vi "stabilizePress_08.vi"() -> ()   [LabVIEW 2011]
uses:
  <vilib>/Analysis/NI_AALPro.lvlib
panel:
  out "Pset array":dbl[](array[numeric])
  out "Pset array":dbl[](array[numeric])
  in  "max plot points":i32=60
  in  "max poly order":u16=2
  out "tune setpoint":dbl=9.864666666660924
  in  "points to fit":i32=4
  out "dt_array":dbl[](array[numeric])
  out "P_i+1 (torr)":dbl caption="predicted next P (torr)" format="%.2f"
  out "Polynomial Coefficients":dbl[](array[numeric])
  in  "polynomial order":dbl=2.0
  out "P array":dbl[](array[numeric])
  out "t array":dbl[](array[numeric])
  in  "i":u16=11
  out "tElaps":dbl=14.796999999991385
  in  "dT_fit(s)":dbl=0.5
  in  "tTotal(s)":dbl=30.0
  out "XY Graph":cluster{"Value":dbl[], "Value":dbl[]}[](graph)
  out "stabilize done":bool
  in  "tExp(s)":dbl=15.0
  out "Set Point (torr)":dbl=20.0 format="%.2f"
  out "Setpoint Index":string="C"
  out "Setpoint Index control":u16(ring)=2 caption="Setpoint" items=["A", "B", "C", "D"]
  out "t_0":dbl=69652.793
  in  "time done (s)":dbl
  out "Wait to set":bool
  out "IO error":errorcluster={"status"=FALSE, "code"=1073676418, "source"="VISA Close in WriteAdaptorr04.vi->writeSetPoint_01.vi->stabilizePress_05.vi"}
  in  "stop":bool=TRUE
  out "Pi (torr)":dbl=6.790000000000001 caption="P(torr)" format="%.2f"
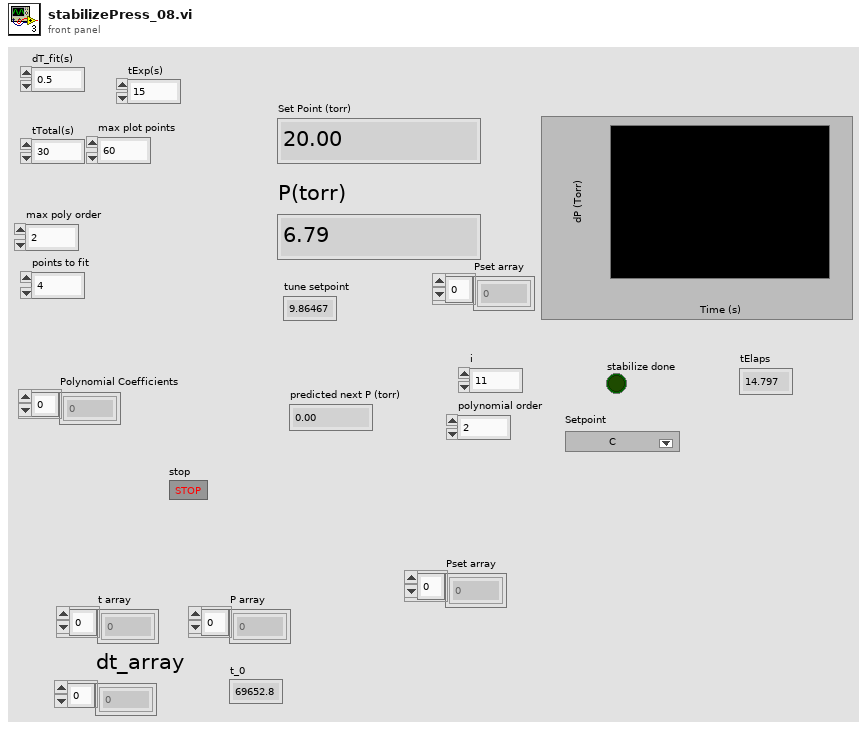
[diagram p1: front panel]
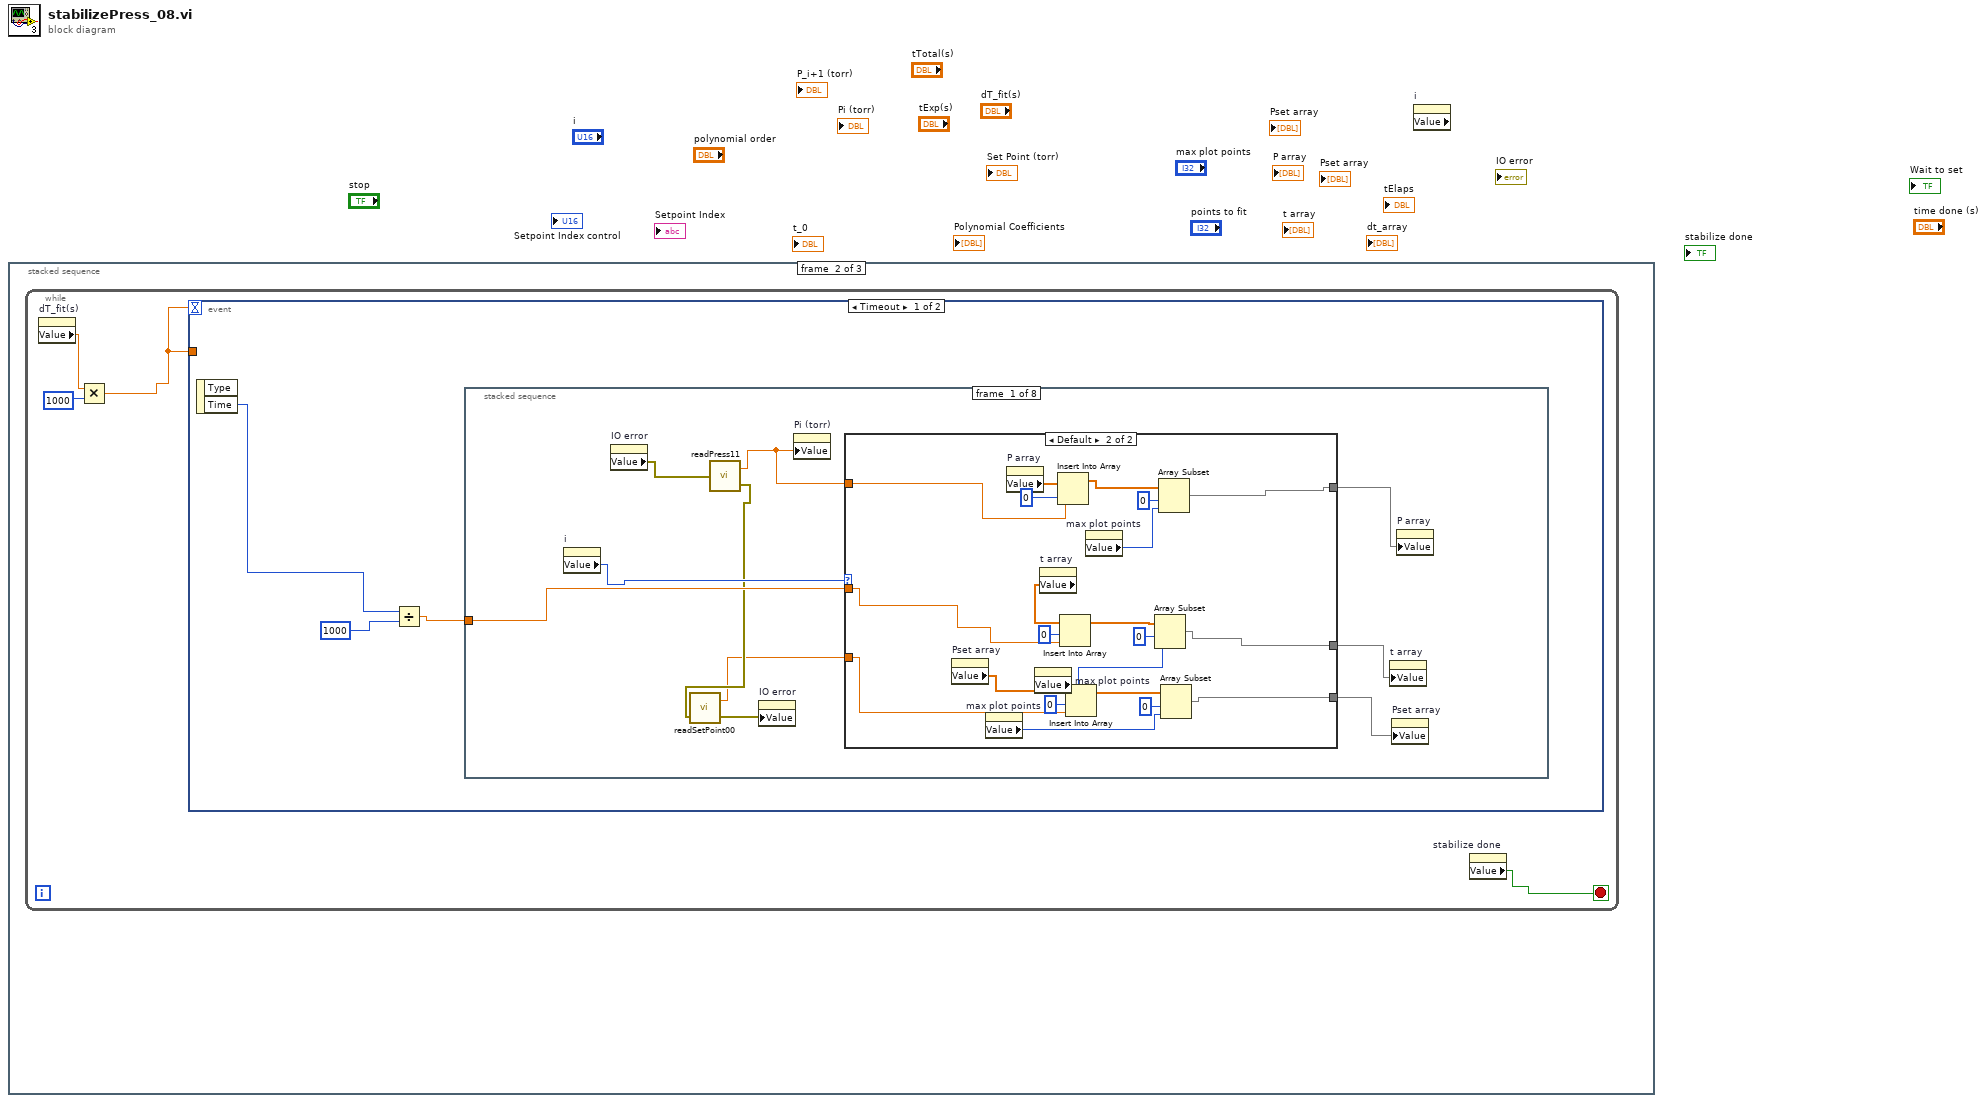
[diagram p0: block diagram]
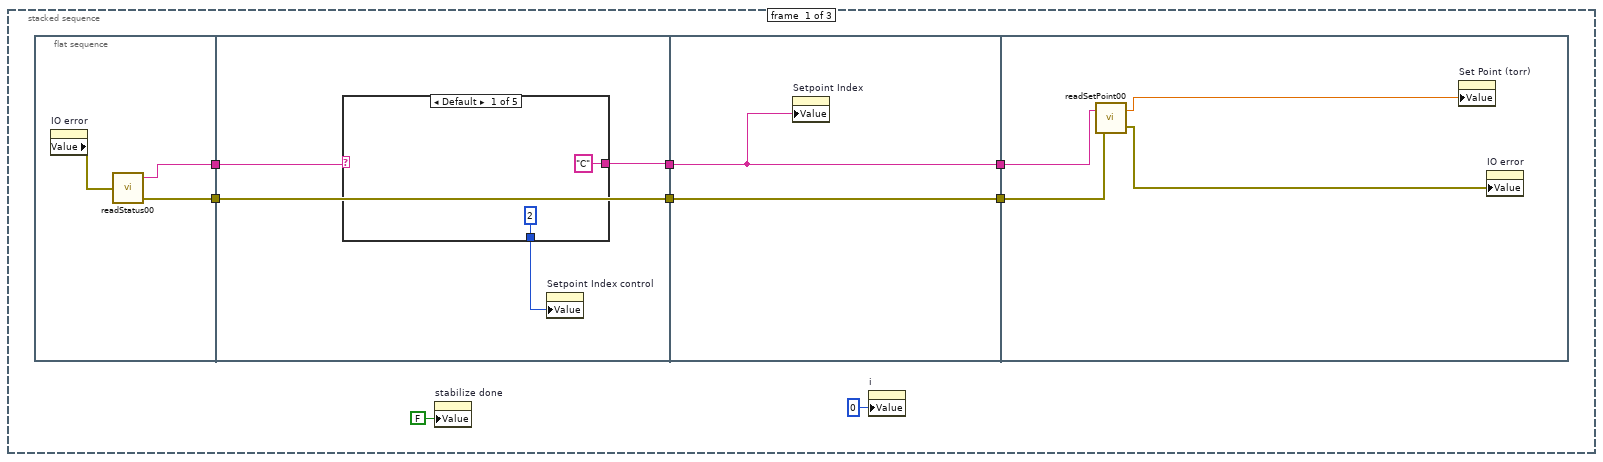
[diagram p2: hidden frame]
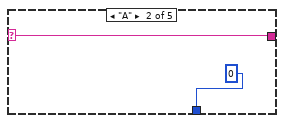
[diagram p3: hidden frame]
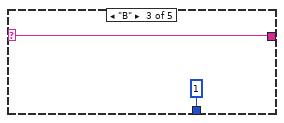
[diagram p4: hidden frame]
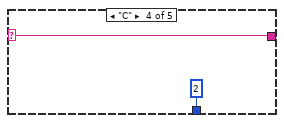
[diagram p5: hidden frame]
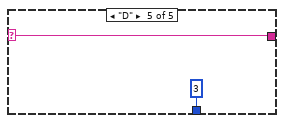
[diagram p6: hidden frame]
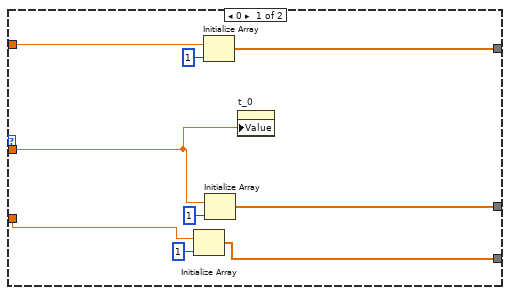
[diagram p7: hidden frame]
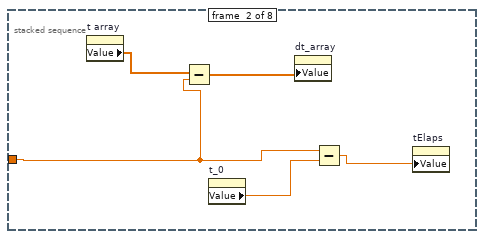
[diagram p8: hidden frame]
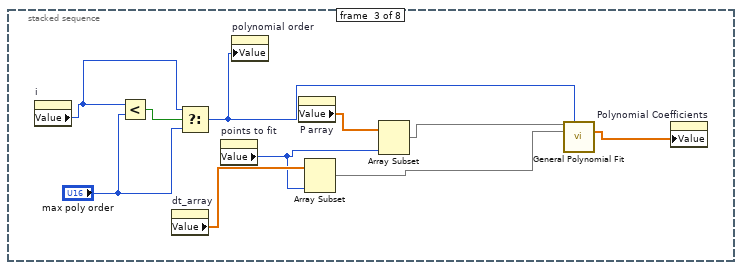
[diagram p9: hidden frame]
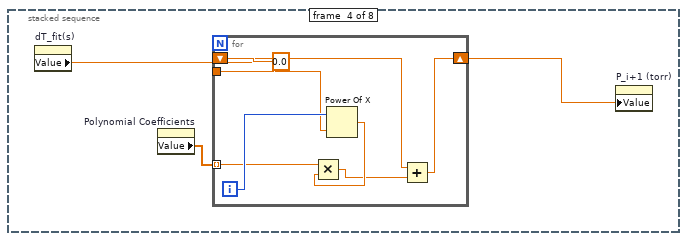
[diagram p10: hidden frame]
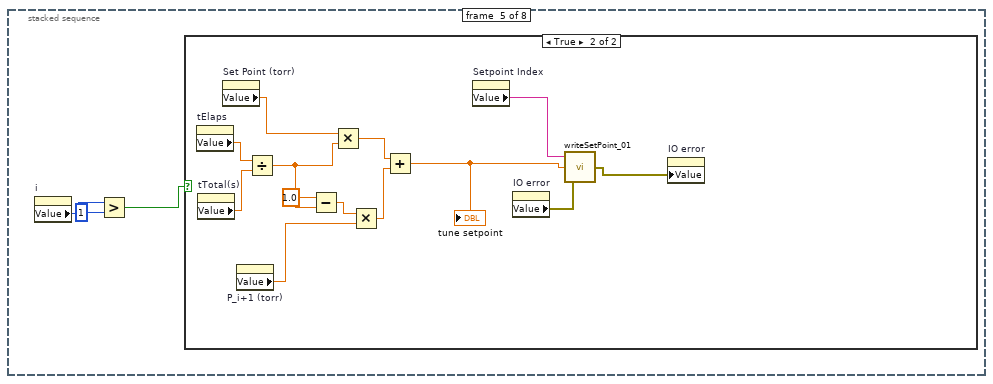
[diagram p11: hidden frame]
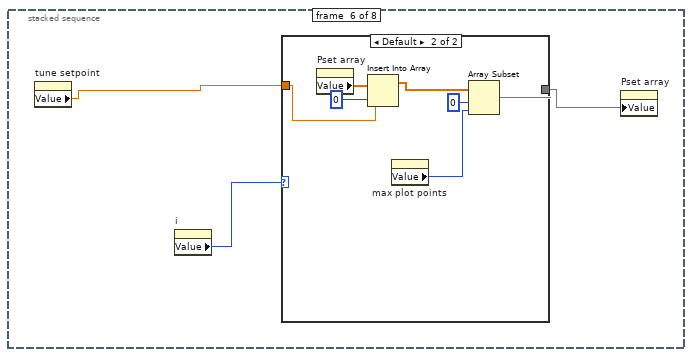
[diagram p13: hidden frame]
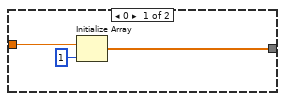
[diagram p14: hidden frame]
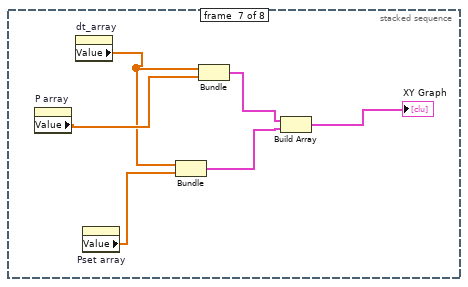
[diagram p15: hidden frame]
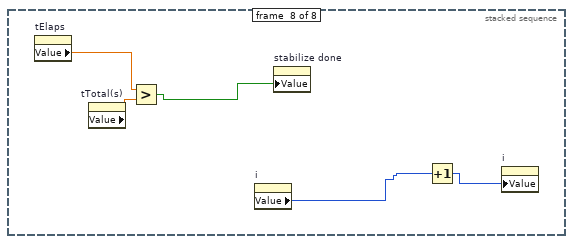
[diagram p16: hidden frame]
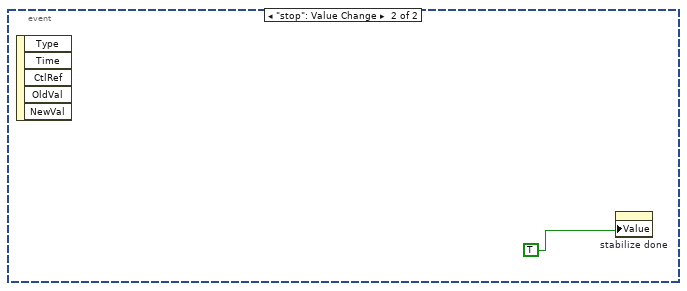
[diagram p17: hidden frame]
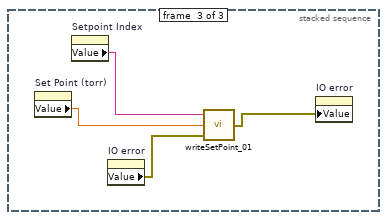
[diagram p18: hidden frame]
diagram:
  n1 = stacked-sequence {
    frame #0 {
      n2 = flat-sequence {
        tunnel: [w10] -> w8
        tunnel: [w9] -> w7
        tunnel: w8 -> [w14]
        tunnel: [w13] -> w6
        tunnel: w7 -> [w15]
        tunnel: [w15] -> w5
        tunnel: w6 -> [w26]
        tunnel: [w26] -> w4
        tunnel: w5 -> [w27]
        tunnel: [w27] -> w3
        tunnel: w4 -> [w31]
        tunnel: w3 -> [w30]
        frame #0 {
          n3 = property on="IO error" class="Clust (strict)"() -> ("Value"=w11:errorcluster)  [unwired: 2 in, 2 out]
          n4 = call "readStatus00.vi"("error in"=w11) -> ("Setpoint"=w10:string, "error out"=w9:errorcluster)  [unwired: 1 out]
        }
        frame #1 {
          n5 = case shown="Default" w14 {
            selector: w14 -> [_ w19 w20 w22 w24]
            tunnel: ["C" w19 w20 w22 w24] -> w13
            tunnel: [u16 2 ("Ring") u16 0 ("Ring") u16 1 ("Ring") u16 2 ("Ring") u16 3 ("Ring")] -> w12
            frame Default {
            }
            frame "A" {
            }
            frame "B" {
            }
            frame "C" {
            }
            frame "D" {
            }
          }
          n6 = property on="Setpoint Index control" class="Ring (strict)"("Value"=w12) -> ()  [unwired: 2 in, 2 out]
        }
        frame #2 {
          n7 = property on="Setpoint Index" class="Str"("Value"=w26) -> ()  [unwired: 2 in, 2 out]
        }
        frame #3 {
          n8 = call "readSetPoint00.vi"("error in"=w30, "Setpoint"=w31) -> ("error out"=w29:errorcluster, "P"=w28:dbl)
          n9 = property on="Set Point (torr)" class="DigNum (strict)"("Value"=w28) -> ()  [unwired: 2 in, 2 out]
          n10 = property on="IO error" class="Clust (strict)"("Value"=w29) -> ()  [unwired: 2 in, 2 out]
        }
      }
      n11 = property on="stabilize done" class="Bool (strict)"("Value"=FALSE ("fit done")) -> ()  [unwired: 2 in, 2 out]
      n12 = property on="i" class="DigNum (strict)"("Value"=u16 0 ("i")) -> ()  [unwired: 2 in, 2 out]
    }
    frame #1 {
      n13 = while {
        stop <- w33 stop-if-true
        n14 = property on="dT_fit(s)" class="DigNum (strict)"() -> ("Value"=w34:dbl)  [unwired: 2 in, 2 out]
        n15 = Multiply(x=w34, y=u32 1000) -> (x*y=w32:dbl)
        n16 = event shown="[0] Timeout" {
          selector: _ -> [_ _]
          dyn-events: _ -> [_ _]
          timeout: w32 -> [_ _]
          tunnel: w32 -> [_ _]
          event Timeout {
            n17 = event-data() -> ("Time"=w36:u32)  [unwired: 1 in, 1 out]
            n18 = Divide(x=w36, y=i64 1000) -> (x/y=w37:dbl)
            n19 = stacked-sequence {
              tunnel: w37 -> [w43 w81 _ _ _ _ _ _]
              frame #0 {
                n20 = property on="i" class="DigNum (strict)"() -> ("Value"=w47:u16)  [unwired: 2 in, 2 out]
                n21 = property on="IO error" class="Clust (strict)"() -> ("Value"=w48:errorcluster)  [unwired: 2 in, 2 out]
                n22 = call "readPress11.vi"("error in"=w48) -> ("P"=w46:dbl, "error out"=w42:errorcluster)
                n23 = call "readSetPoint00.vi"("error in"=w42) -> ("error out"=w41:errorcluster, "P"=w40:dbl)  [unwired: 1 in]
                n24 = property on="IO error" class="Clust (strict)"("Value"=w41) -> ()  [unwired: 2 in, 2 out]
                n25 = property on="Pi (torr)" class="DigNum (strict)"("Value"=w46) -> ()  [unwired: 2 in, 2 out]
                n26 = case shown="Default" w47 {
                  tunnel: w43 -> [w52 w69]
                  tunnel: w46 -> [w56 w78]
                  tunnel: [w54 w71] -> w45
                  tunnel: [w53 w70] -> w44
                  tunnel: w40 -> [w50 w62]
                  tunnel: [w49 w60] -> w39
                  frame 0 {
                    n27 = Initialize Array(w50, 1 ("dimension size")) -> (w49:dbl[])
                    n28 = Initialize Array(w56, 1 ("dimension size")) -> (w54:dbl[])
                    n29 = Initialize Array(w52, 1 ("dimension size")) -> (w53:dbl[])
                    n30 = property on="t_0" class="DigNum (strict)"("Value"=w52) -> ()  [unwired: 2 in, 2 out]
                  }
                  frame Default {
                    n31 = property on="Pset array" class="Arr (strict)"() -> ("Value"=w59:dbl[])  [unwired: 2 in, 2 out]
                    n32 = property on="max plot points" class="DigNum (strict)"() -> ("Value"=w58:i32)  [unwired: 2 in, 2 out]
                    n33 = property on="P array" class="Arr (strict)"() -> ("Value"=w77:dbl[])  [unwired: 2 in, 2 out]
                    n34 = property on="max plot points" class="DigNum (strict)"() -> ("Value"=w65:i32)  [unwired: 2 in, 2 out]
                    n35 = property on="t array" class="Arr (strict)"() -> ("Value"=w76:dbl[])  [unwired: 2 in, 2 out]
                    n36 = Insert Into Array(array=w77, index=0, new element=w78) -> (w75:dbl[])
                    n37 = Insert Into Array(array=w76, index=0, new element=w69) -> (w73:dbl[])
                    n38 = Insert Into Array(array=w59, index=0, new element=w62) -> (w61:dbl[])
                    n39 = property on="max plot points" class="DigNum (strict)"() -> ("Value"=w66:i32)  [unwired: 2 in, 2 out]
                    n40 = Array Subset(array=w73, index=0, length=w65) -> (w70:dbl[])
                    n41 = Array Subset(array=w75, index=0, length=w66) -> (w71:dbl[])
                    n42 = Array Subset(array=w61, index=0, length=w58) -> (w60:dbl[])
                  }
                }
                n43 = property on="t array" class="Arr (strict)"("Value"=w44) -> ()  [unwired: 2 in, 2 out]
                n44 = property on="Pset array" class="Arr (strict)"("Value"=w39) -> ()  [unwired: 2 in, 2 out]
                n45 = property on="P array" class="Arr (strict)"("Value"=w45) -> ()  [unwired: 2 in, 2 out]
              }
              frame #1 {
                n46 = property on="t array" class="Arr (strict)"() -> ("Value"=w82:dbl[])  [unwired: 2 in, 2 out]
                n47 = Subtract(x=w82, y=w81) -> (x-y=w83:dbl[])
                n48 = property on="t_0" class="DigNum (strict)"() -> ("Value"=w80:dbl)  [unwired: 2 in, 2 out]
                n49 = property on="dt_array" class="Arr (strict)"("Value"=w83) -> ()  [unwired: 2 in, 2 out]
                n50 = Subtract(x=w81, y=w80) -> (x-y=w79:dbl)
                n51 = property on="tElaps" class="DigNum (strict)"("Value"=w79) -> ()  [unwired: 2 in, 2 out]
              }
              frame #2 {
                n52 = property on="i" class="DigNum (strict)"() -> ("Value"=w90:u16)  [unwired: 2 in, 2 out]
                n53 = Less?(x=w90, y="max poly order") -> (x < y?=w93:bool)
                n54 = property on="dt_array" class="Arr (strict)"() -> ("Value"=w88:dbl[])  [unwired: 2 in, 2 out]
                n55 = Select(t=w90, s=w93, f="max poly order") -> (s? t:f=w91:u16)
                n56 = property on="points to fit" class="DigNum (strict)"() -> ("Value"=w85:i32)  [unwired: 2 in, 2 out]
                n57 = property on="polynomial order" class="DigNum (strict)"("Value"=w91) -> ()  [unwired: 2 in, 2 out]
                n58 = property on="P array" class="Arr (strict)"() -> ("Value"=w86:dbl[])  [unwired: 2 in, 2 out]
                n59 = Array Subset(array=w88, length=w85) -> (w87:dbl[])  [unwired: 1 in]
                n60 = Array Subset(array=w86, length=w85) -> (w84:dbl[])  [unwired: 1 in]
                n61 = call <vilib>:"General Polynomial Fit.vi"("Y"=w84, "polynomial order"=w91, "X"=w87) -> ("Polynomial Coefficients"=w92:dbl[])  [unwired: 9 in, 3 out]
                n62 = property on="Polynomial Coefficients" class="Arr (strict)"("Value"=w92) -> ()  [unwired: 2 in, 2 out]
              }
              frame #3 {
                n63 = property on="dT_fit(s)" class="DigNum (strict)"() -> ("Value"=w95:dbl)  [unwired: 2 in, 2 out]
                n64 = property on="Polynomial Coefficients" class="Arr (strict)"() -> ("Value"=w97:dbl[])  [unwired: 2 in, 2 out]
                n65 = for {
                  tunnel: w95 -> [w103]
                  tunnel: w97 -> [w102] mode=indexing
                  shift-right: [w98] -> w94
                  shift-left: 0.0 -> [w99]
                  i -> [w104]
                  n66 = Power Of X(1:w103, 2:w104) -> (0:w101:dbl)
                  n67 = Multiply(x=w102, y=w101) -> (x*y=w100:dbl)
                  n68 = Add(x=w99, y=w100) -> (x+y=w98:dbl)
                }
                n69 = property on="P_i+1 (torr)" class="DigNum (strict)"("Value"=w94) -> ()  [unwired: 2 in, 2 out]
              }
              frame #4 {
                n70 = property on="i" class="DigNum (strict)"() -> ("Value"=w107:u16)  [unwired: 2 in, 2 out]
                n71 = Greater?(x=w107, y=u16 1) -> (0:w105:bool)
                n72 = case shown="True" w105 {
                  frame False {
                  }
                  frame True {
                    n73 = property on="tElaps" class="DigNum (strict)"() -> ("Value"=w117:dbl)  [unwired: 2 in, 2 out]
                    n74 = property on="tTotal(s)" class="DigNum (strict)"() -> ("Value"=w116:dbl)  [unwired: 2 in, 2 out]
                    n75 = property on="Set Point (torr)" class="DigNum (strict)"() -> ("Value"=w115:dbl)  [unwired: 2 in, 2 out]
                    n76 = property on="P_i+1 (torr)" class="DigNum (strict)"() -> ("Value"=w110:dbl)  [unwired: 2 in, 2 out]
                    n77 = Divide(x=w117, y=w116) -> (x/y=w113:dbl)
                    n78 = Subtract(x=1.0, y=w113) -> (x-y=w111:dbl)
                    n79 = Multiply(x=w115, y=w113) -> (x*y=w114:dbl)
                    n80 = Multiply(x=w111, y=w110) -> (x*y=w109:dbl)
                    n81 = Add(x=w114, y=w109) -> (x+y=w108:dbl)
                    "tune setpoint" <- w108
                    n82 = property on="Setpoint Index" class="Str"() -> ("Value"=w120:string)  [unwired: 2 in, 2 out]
                    n83 = property on="IO error" class="Clust (strict)"() -> ("Value"=w119:errorcluster)  [unwired: 2 in, 2 out]
                    n84 = call "writeSetPoint_01.vi"("error in"=w119, "P (Torr)"=w108, "Setpoint"=w120) -> ("error out"=w118:errorcluster)
                    n85 = property on="IO error" class="Clust (strict)"("Value"=w118) -> ()  [unwired: 2 in, 2 out]
                  }
                }
              }
              frame #5 {
                n86 = property on="tune setpoint" class="DigNum (strict)"() -> ("Value"=w121:dbl)  [unwired: 2 in, 2 out]
                n87 = property on="i" class="DigNum (strict)"() -> ("Value"=w123:u16)  [unwired: 2 in, 2 out]
                n88 = case shown="Default" w123 {
                  tunnel: w121 -> [w126 w133]
                  tunnel: [w124 w129] -> w122
                  frame 0 {
                    n89 = Initialize Array(w126, 1 ("dimension size")) -> (w124:dbl[])
                  }
                  frame Default {
                    n90 = property on="Pset array" class="Arr (strict)"() -> ("Value"=w132:dbl[])  [unwired: 2 in, 2 out]
                    n91 = Insert Into Array(array=w132, index=0, new element=w133) -> (w131:dbl[])
                    n92 = property on="max plot points" class="DigNum (strict)"() -> ("Value"=w127:i32)  [unwired: 2 in, 2 out]
                    n93 = Array Subset(array=w131, index=0, length=w127) -> (w129:dbl[])
                  }
                }
                n94 = property on="Pset array" class="Arr (strict)"("Value"=w122) -> ()  [unwired: 2 in, 2 out]
              }
              frame #6 {
                n95 = property on="P array" class="Arr (strict)"() -> ("Value"=w139:dbl[])  [unwired: 2 in, 2 out]
                n96 = property on="dt_array" class="Arr (strict)"() -> ("Value"=w138:dbl[])  [unwired: 2 in, 2 out]
                n97 = property on="Pset array" class="Arr (strict)"() -> ("Value"=w137:dbl[])  [unwired: 2 in, 2 out]
                n98 = Bundle "Bundle"("Value"=w138, "Value"=w137) -> (w135:cluster{"Value":dbl[], "Value":dbl[]})  [unwired: 1 in]
                n99 = Bundle "Bundle"("Value"=w138, "Value"=w139) -> (w136:cluster{"Value":dbl[], "Value":dbl[]})  [unwired: 1 in]
                n100 = Build Array "Build Array"(w136, w135) -> (→"XY Graph":cluster{"Value":dbl[], "Value":dbl[]}[])
              }
              frame #7 {
                n101 = property on="tElaps" class="DigNum (strict)"() -> ("Value"=w140:dbl)  [unwired: 2 in, 2 out]
                n102 = property on="tTotal(s)" class="DigNum (strict)"() -> ("Value"=w144:dbl)  [unwired: 2 in, 2 out]
                n103 = Greater?(x=w140, y=w144) -> (0:w143:bool)
                n104 = property on="i" class="DigNum (strict)"() -> ("Value"=w141:u16)  [unwired: 2 in, 2 out]
                n105 = property on="stabilize done" class="Bool (strict)"("Value"=w143) -> ()  [unwired: 2 in, 2 out]
                n106 = Increment(x=w141) -> (x+1=w142:u16)
                n107 = property on="i" class="DigNum (strict)"("Value"=w142) -> ()  [unwired: 2 in, 2 out]
              }
            }
          }
          event "stop": Value Change {
            n108 = event-data() -> ()  [unwired: 1 in, 5 out]
            n109 = property on="stabilize done" class="Bool (strict)"("Value"=TRUE ("stabilize done")) -> ()  [unwired: 2 in, 2 out]
          }
        }
        n110 = property on="stabilize done" class="Bool (strict)"() -> ("Value"=w33:bool)  [unwired: 2 in, 2 out]
      }
    }
    frame #2 {
      n111 = property on="Set Point (torr)" class="DigNum (strict)"() -> ("Value"=w149:dbl)  [unwired: 2 in, 2 out]
      n112 = property on="Setpoint Index" class="Str"() -> ("Value"=w148:string)  [unwired: 2 in, 2 out]
      n113 = property on="IO error" class="Clust (strict)"() -> ("Value"=w147:errorcluster)  [unwired: 2 in, 2 out]
      n114 = call "writeSetPoint_01.vi"("error in"=w147, "P (Torr)"=w149, "Setpoint"=w148) -> ("error out"=w146:errorcluster)
      n115 = property on="IO error" class="Clust (strict)"("Value"=w146) -> ()  [unwired: 2 in, 2 out]
    }
  }
  n116 = property on="i" class="DigNum (strict)" props=["Value"]() -> ()  [unwired: 2 in, 3 out]
